vi "Time to Number.vi"(4 "time stamp":timestamp) -> (0 "time (s)":dbl format="%#_24g", 1 "time (h.mm)":dbl)   [LabVIEW 2009]
doc: "Takes a time stamp as an input and converts it to decimal time in the format h.mm, as well as to fractional seconds since Friday, January 1, 1904, Universal Time."
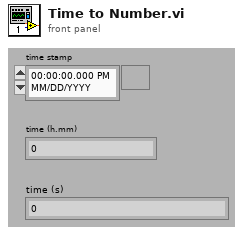
[diagram p1: front panel]
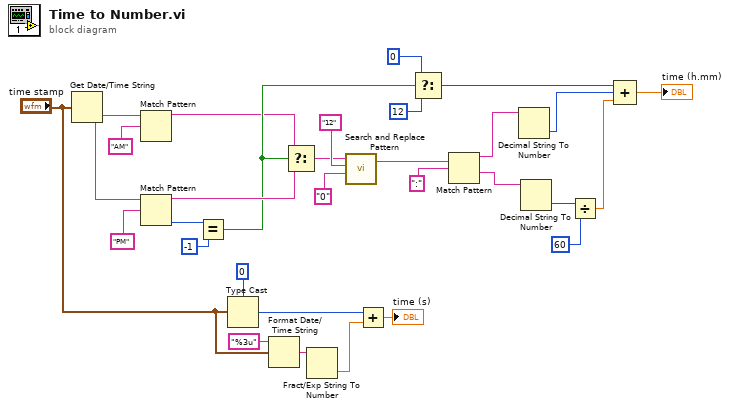
[diagram p0: block diagram]
diagram:
  n1 = Get Date/Time String(seconds (now)="time stamp") -> (time string=w29:string)  [unwired: 3 out]
  n2 = Match Pattern(string=w29, regular expression="AM") -> (before substring=w8:string)  [unwired: 4 out]
  n3 = Match Pattern(string=w29, regular expression="PM") -> (before substring=w14:string, offset past match=w15:i32)  [unwired: 3 out]
  n4 = Equal?(x=w15, y=-1) -> (x = y?=w11:bool)
  n5 = Type Cast(type=u64 0, x="time stamp") -> (*(type *) &x=w4:u64)
  n6 = Format Date/Time String(time format string (%c)="%3u", seconds (now)="time stamp") -> (date/time string=w5:string)  [unwired: 1 out]
  n7 = Select(t=w8, s=w11, f=w14) -> (s? t:f=w10:string)
  n8 = Fract/Exp String To Number(string=w5) -> (number=w3:dbl)  [unwired: 4 out]
  n9 = call <vilib>:"Search and Replace Pattern.vi"("string"=w10, "regular expression (\"\")"="12", "replace string (\"\")"="0") -> ("result string"=w9:string)  [unwired: 3 out]
  n10 = Add(x=w4, y=w3) -> (x+y=→"time (s)":dbl)
  n11 = Select(t=0, s=w11, f=12) -> (s? t:f=w17:i32)
  n12 = Match Pattern(string=w9, regular expression=":") -> (before substring=w23:string, after substring=w22:string)  [unwired: 3 out]
  n13 = Decimal String To Number(string=w23) -> (number=w20:i32)  [unwired: 3 out]
  n14 = Decimal String To Number(string=w22) -> (number=w19:i32)  [unwired: 3 out]
  n15 = Divide(x=w19, y=60) -> (x/y=w18:dbl)
  n16 = Compound Arithmetic op=ADD(w17, w20, w18) -> (→"time (h.mm)":dbl)
